vi "StringDatetimeToDateAndTimeString.vi"(10 "String":string) -> (0 "time stamp":timestamp, 1 "Time String":string, 3 "Date String":string)   [LabVIEW 2012]
uses:
  <vilib>/Utility/miscctls.llb/LVDateTimeRec.ctl
panel:
  out "output cluster":T1
  in  "date time rec":T1
  in  "date time rec 2":T1
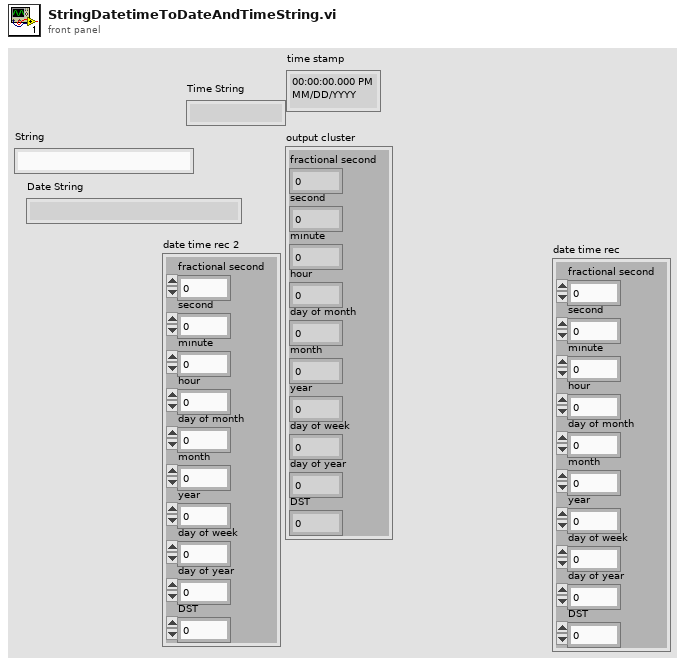
[diagram p1: front panel]
types:
  T1 = typedef "LVDateTimeRec.ctl" = cluster{"fractional second":dbl, "second":i32, "minute":i32, "hour":i32, "day of month":i32, "month":i32, "year":i32, "day of week":i32, "day of year":i32, "DST":i32}
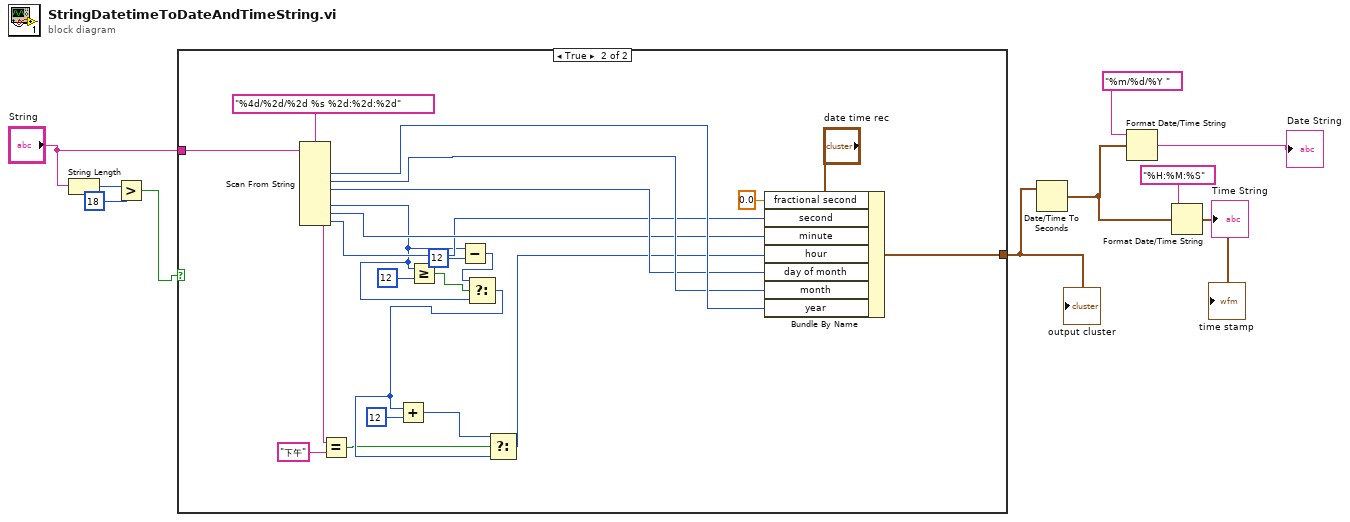
[diagram p0: block diagram]
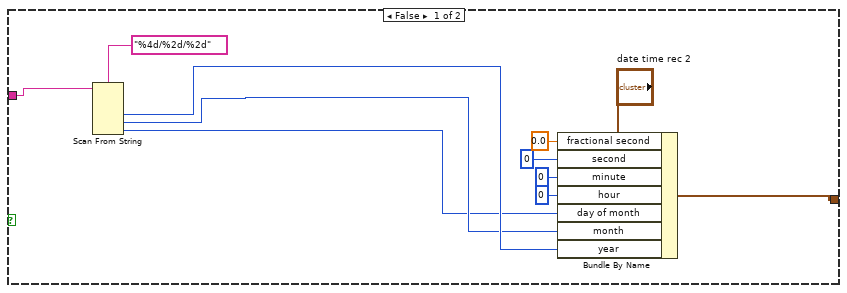
[diagram p2: hidden frame]
diagram:
  n1 = String Length(string="String") -> (length=w10:i32)
  n2 = Greater?(x=w10, y=18) -> (0:w8:bool)
  n3 = case shown="True" w8 {
    tunnel: "String" -> [w15 w30]
    tunnel: [w11 w29] -> w6
    frame False {
      n4 = Scan From String(format string="%4d/%2d/%2d", input string=w15) -> (output 1=w18:i32, output 2=w17:i32, output 3=w16:i32)  [unwired: 5 in, 3 out]
      n5 = Bundle By Name(cluster="date time rec 2", "fractional second"=0.0, "second"=0, "minute"=0, "hour"=0, "day of month"=w16, "month"=w17, "year"=w18) -> (w11:T1)
    }
    frame True {
      n6 = Scan From String(format string="%4d/%2d/%2d %s %2d:%2d:%2d", input string=w30) -> (output 1=w36:i32, output 2=w35:i32, output 3=w34:i32, output 4=w42:string, output 5=w26:i32, output 6=w32:i32, output 7=w31:i32)  [unwired: 9 in, 3 out]
      n7 = Equal?(x=w42, y="下午") -> (x = y?=w22:bool)
      n8 = Greater Or Equal?(x=w26, y=12) -> (x >= y?=w27:bool)
      n9 = Subtract(x=w26, y=12) -> (x-y=w24:i32)
      n10 = Select(t=w24, s=w27, f=w26) -> (s? t:f=w23:i32)
      n11 = Add(x=w23, y=12) -> (x+y=w39:i32)
      n12 = Select(t=w39, s=w22, f=w23) -> (s? t:f=w33:i32)
      n13 = Bundle By Name(cluster="date time rec", "fractional second"=0.0, "second"=w31, "minute"=w32, "hour"=w33, "day of month"=w34, "month"=w35, "year"=w36) -> (w29:T1)
    }
  }
  "output cluster" <- w6
  n14 = Date/Time To Seconds(2:w6) -> (0:w3:timestamp)  [unwired: 1 in]
  "time stamp" <- w3
  n15 = Format Date/Time String(time format string (%c)="%m/%d/%Y ", seconds (now)=w3) -> (date/time string=→"Date String":string)  [unwired: 1 in]
  n16 = Format Date/Time String(time format string (%c)="%H:%M:%S", seconds (now)=w3) -> (date/time string=→"Time String":string)  [unwired: 1 in]
